vi "csm_lumikki_instron_initRamp.vi"(10 "rampRate":dbl, 11 "rampAmplitude":dbl) -> (1 "startSetRampOut":bool, 2 "rampRateOut":dbl, 3 "rampAmplitudeOut":dbl)   [LabVIEW 2009]
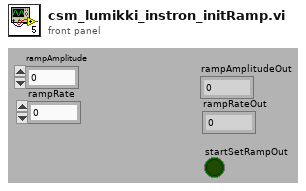
[diagram p1: front panel]
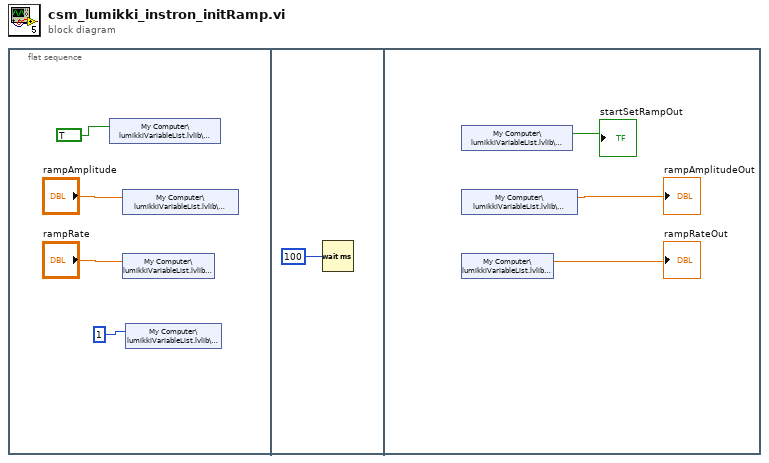
[diagram p0: block diagram]
diagram:
  n1 = flat-sequence {
    frame #0 {
      n2 = shared-variable "My Computer\\lumikkiVariableList.lvlib\\startSetRamp"(TRUE ("Busy")) -> ()  [unwired: 1 in, 1 out]
      n3 = shared-variable "My Computer\\lumikkiVariableList.lvlib\\rampAmplitude"("rampAmplitude") -> ()  [unwired: 1 in, 1 out]
      n4 = shared-variable "My Computer\\lumikkiVariableList.lvlib\\rampRate"("rampRate") -> ()  [unwired: 1 in, 1 out]
      n5 = shared-variable "My Computer\\lumikkiVariableList.lvlib\\channelInt"(1 ("channelInt")) -> ()  [unwired: 1 in, 1 out]
    }
    frame #1 {
      n6 = Wait (ms)(milliseconds to wait=u32 100) -> ()  [unwired: 1 out]
    }
    frame #2 {
      n7 = shared-variable "My Computer\\lumikkiVariableList.lvlib\\startSetRamp"() -> (→"startSetRampOut":bool)  [unwired: 1 in, 1 out]
      n8 = shared-variable "My Computer\\lumikkiVariableList.lvlib\\rampAmplitude"() -> (→"rampAmplitudeOut":dbl)  [unwired: 1 in, 1 out]
      n9 = shared-variable "My Computer\\lumikkiVariableList.lvlib\\rampRate"() -> (→"rampRateOut":dbl)  [unwired: 1 in, 1 out]
    }
  }
